vi "TangoAttributeConfigEventTest.vi"() -> ()   [LabVIEW 2013, in "examples.lvlib"]
uses:
  examples.lvlib
  vis/lv-2013/tango_vi.llb/tango.lvlib
panel:
  out "Attr: double_scalar":T1
  out "Attr: long_scalar":T1
  out "?":string="\n1. Be sure your TangoTest  device is running \n\n2. Open Jive in read/write mode\n\n3. Click on the 'Device' tab \n\n4. Locate your TangoTest devicein the devices tree\n\n5. Expand  the corresponding entry \n\n6. Click on 'Attribute config'\n\n7. Change any component of the configuration of the'long_scalar' or 'double_scalar' attribute\n\n8. This LabVIEW example should receive a notification of  modification"
  in  "?":bool
  in  "TangoTest Device Name":string="sys/tg_test/1"
  # "TANGO \"ATTRIBUTE CONFIG CHANGED\" EVENT DEMO"
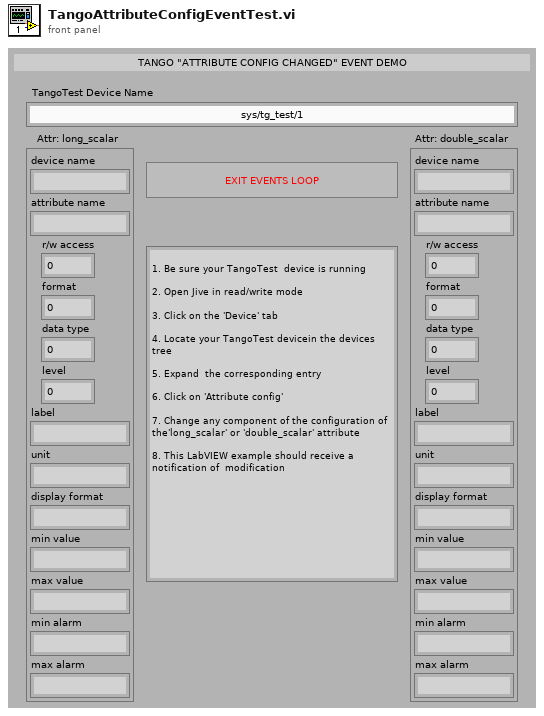
[diagram p1: front panel]
types:
  T1 = cluster{"device name":string, "attribute name":string, "r/w access":i16, "format":i16, "data type":i16, "level":i16, "label":string, "unit":string, "display format":string, "min value":string, "max value":string, "min alarm":string, "max alarm":string}
  T2 = cluster{"user event ref":refnum<user-event>, "user event reg refnum":refnum<event-registration>}
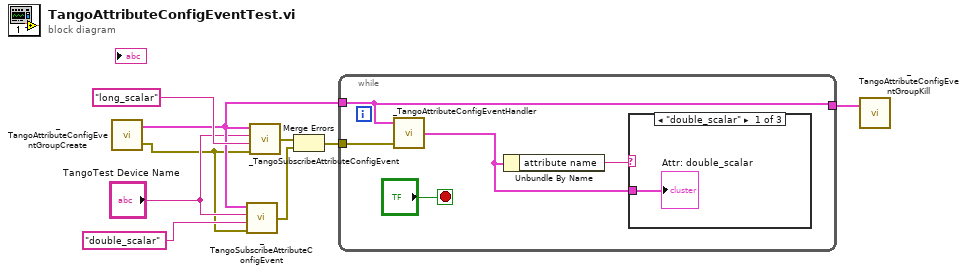
[diagram p0: block diagram]
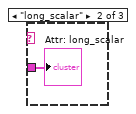
[diagram p2: hidden frame]
diagram:
  n1 = call "_TangoAttributeConfigEventGroupCreate.vi"() -> ("attribute config event ref"=w7:T2, "error out"=w4:errorcluster)  [unwired: 1 in]
  n2 = call "_TangoSubscribeAttributeConfigEvent.vi"("error in"=w4, "attribute name"="double_scalar", "device name"="TangoTest Device Name", "attribute config event ref"=w7) -> ("error out"=w2:errorcluster)
  n3 = call "_TangoSubscribeAttributeConfigEvent.vi"("error in"=w4, "attribute name"="long_scalar", "device name"="TangoTest Device Name", "attribute config event ref"=w7) -> ("error out"=w3:errorcluster)
  n4 = Merge Errors(w3, w2) -> (w1:errorcluster)
  n5 = while {
    tunnel: w7 -> [w13]
    tunnel: w1 -> [w14]
    tunnel: [w13] -> w8
    stop <- "?" stop-if-true
    n6 = call "_TangoAttributeConfigEventHandler.vi"("error in"=w14, "attribute config event ref"=w13) -> ("attribute info"=w10:T1)  [unwired: 1 in, 2 out]
    n7 = Unbundle By Name(w10) -> ("attribute name"=w11:string)
    n8 = case shown="\"double_scalar\"" w11 {
      tunnel: w10 -> [w15 w16 _]
      frame "double_scalar" {
        "Attr: double_scalar" <- w15
      }
      frame "long_scalar" {
        "Attr: long_scalar" <- w16
      }
      frame Default {
      }
    }
  }
  n9 = call "_TangoAttributeConfigEventGroupKill.vi"("attribute config event ref"=w8) -> ()  [unwired: 1 in, 1 out]
